vi "View param.vi"() -> ()   [LabVIEW 2019]
uses:
  Database/Progress.vi
panel:
  in  "PARNames":refnum<data-value>
  in  "PAR":refnum<data-value>
  in  "PARsh":refnum<data-value>
  in  "PAR_I":refnum<data-value>
  out "HandlingView":bool[](array[boolean])
  out "error out":errorcluster
  in  "n_elem2":i32
  in  "conninfo":T1={"host"="localhost", "port"="5432", "client_encoding"="WIN1251", "dbname"="system", "user"="postgres", "password"=""}
  in  "parameters 2":string[][](array[string])=[["H1.EB2.1.BT1", "H1.EB2.1.BT3", "H1.EB2.21.BT1", "H1.EB2.22.BT1", "H1.EB2.23.BT1", "H1.EB2.2.BT3", "H1.EB2.BP1", "H1.EB2.EP1.BF1", "H1.EB2.EP1.BT1", "H1.EB2.EP1.BT2", "H1.EB2.QN1", "H1.EP.BP1", "H1.GM2.1.BP1", "H1.GM2.1.HT1.BC1", "H1.GM2.1.HT1.BT1", "H1.GM2.1.QN1", "H1.GM2.2.BP1", "H1.GM2.2.QN1", "H1.GM2.2.QN2", "H1.GM2.2.QN3", "H1.HW2.BT1", "H1.HW2.BT2", "H1.HW2.BT3", "H1.HW2.BT4"]]
  in  "AOParamView":bool
  in  "DOParamView":bool
  out "n_modules":i32
  out "n_connect":i32
  in  "ModuleHandlingView":bool
  in  "ALRhandlingView":bool
  in  "AIParamView":bool
  out "tick out":u32=100 caption="Время цикла основной программы" min=5 max=500 step=1
  out "archiv AI period  out":u32=1000 caption="Период архивирования аналоговых параметров" min=1 max=100000 step=1
  out "archiv DI period  out":u32=1000 caption="Период архивирования дискретных параметров" min=1 max=100000 step=1
  out "modules read period out":u32=100 caption="Период обновления информации из модулей" min=1 max=100000 step=1
  out "Reread out":bool
  in  "modules read period":u32=500 caption="Период обновления информации из модулей" min=1 max=100000 step=1
  in  "ALR write":bool caption="запись аварийных сообщений"
  in  "DI write":bool caption="запись дискретных параметров"
  in  "AI write":bool caption="запись аналоговых параметров"
  in  "T_DB_write":u32(graph) caption="Время записи в БД"
  in  "archiv DI period":u32=1000 caption="Период архивирования дискретных параметров" min=1 max=100000 step=1
  in  "archiv AI period":u32=1000 caption="Период архивирования аналоговых параметров" min=1 max=100000 step=1
  in  "tick":u32=100 caption="Время цикла основной программы" min=5 max=500 step=1
  in  "n_elem":i32(c297)
  out "PAR progress":i32(slide) scale=0.0..100.0
  in  "Reread":bool
  out "units":string[](array[string])
  in  "AI_9":dbl min=1.0 max=10.0 step=1.0 format="%#.1f"
  in  "AI_10":dbl min=20.0 max=60.0 step=1.0 format="%#.1f"
  in  "AI_5":dbl min=10.0 max=1000.0 step=1.0 format="%#.1f"
  in  "AI_6":dbl min=10.0 max=10000.0 step=10.0 format="%#.1f"
  in  "AI_7":dbl min=1.0 max=10.0 step=1.0 format="%#.1f"
  in  "AI_8":dbl min=1.0 max=10.0 step=1.0 format="%#.1f"
  in  "AI_3":dbl min=1.0 max=50.0 step=1.0 format="%#.1f"
  in  "AI_4":dbl min=60000.0 max=300000.0 step=100.0 format="%#.1f"
  in  "AI_2":dbl min=50.0 max=60000.0 step=50.0 format="%#.1f"
  in  "AI_1":dbl min=50.0 max=60000.0 step=50.0 format="%#.1f"
  in  "ActivatePARView":bool
  out "n param":i32
  in  "parameters":string[](array[string])=["H1.EB2.1.BT1", "H1.EB2.1.BT3", "H1.EB2.21.BT1", "H1.EB2.22.BT1", "H1.EB2.23.BT1", "H1.EB2.2.BT3", "H1.EB2.BP1", "H1.EB2.EP1.BF1", "H1.EB2.EP1.BT1", "H1.EB2.EP1.BT2", "H1.EB2.QN1", "H1.EP.BP1", "H1.GM2.1.BP1", "H1.GM2.1.HT1.BC1", "H1.GM2.1.HT1.BT1", "H1.GM2.1.QN1", "H1.GM2.2.BP1", "H1.GM2.2.QN1", "H1.GM2.2.QN2", "H1.GM2.2.QN3", "H1.HW2.BT1", "H1.HW2.BT2", "H1.HW2.BT3", "H1.HW2.BT4"]
  out "This VI":refnum<vi>
  out "Names table":string[](array[string])=["температура нагревателя", "температура газа после ступени", "температура нагревателя", "температура нагревателя", "температура нагревателя", "температура газа после ступени", "давление газа перед нагревателем", "расход охлаждающей воды", "температура на входе", "температура на выходе", "регулятор расхода азота/тех газа", "давление охлаждающей воды на входе в теплообменник", "давление газа перед дозатором", "ток нагревателя", "температура нагревателя", "регулятор расхода азота/водорода (метана)", "давление газа перед дозатором", "регулятор расхода водорода (метана)", "регулятор природного газа", "дозатор жидкостный", "температура газа на входе в смеситель", "температура стенки смесителя 100 мм", "температура стенки смесителя 200 мм", "температура стенки смесителя на вводе CH4"]
  out "parameters1":string[](array[string])=["H1.EB2.1.BT1", "H1.EB2.1.BT3", "H1.EB2.21.BT1", "H1.EB2.22.BT1", "H1.EB2.23.BT1", "H1.EB2.2.BT3", "H1.EB2.BP1", "H1.EB2.EP1.BF1", "H1.EB2.EP1.BT1", "H1.EB2.EP1.BT2", "H1.EB2.QN1", "H1.EP.BP1", "H1.GM2.1.BP1", "H1.GM2.1.HT1.BC1", "H1.GM2.1.HT1.BT1", "H1.GM2.1.QN1", "H1.GM2.2.BP1", "H1.GM2.2.QN1", "H1.GM2.2.QN2", "H1.GM2.2.QN3", "H1.HW2.BT1", "H1.HW2.BT2", "H1.HW2.BT3", "H1.HW2.BT4"]
  # "mS"
  # "из"
  # "подключено"
  # "mS"
  # "mS"
  # "mS"
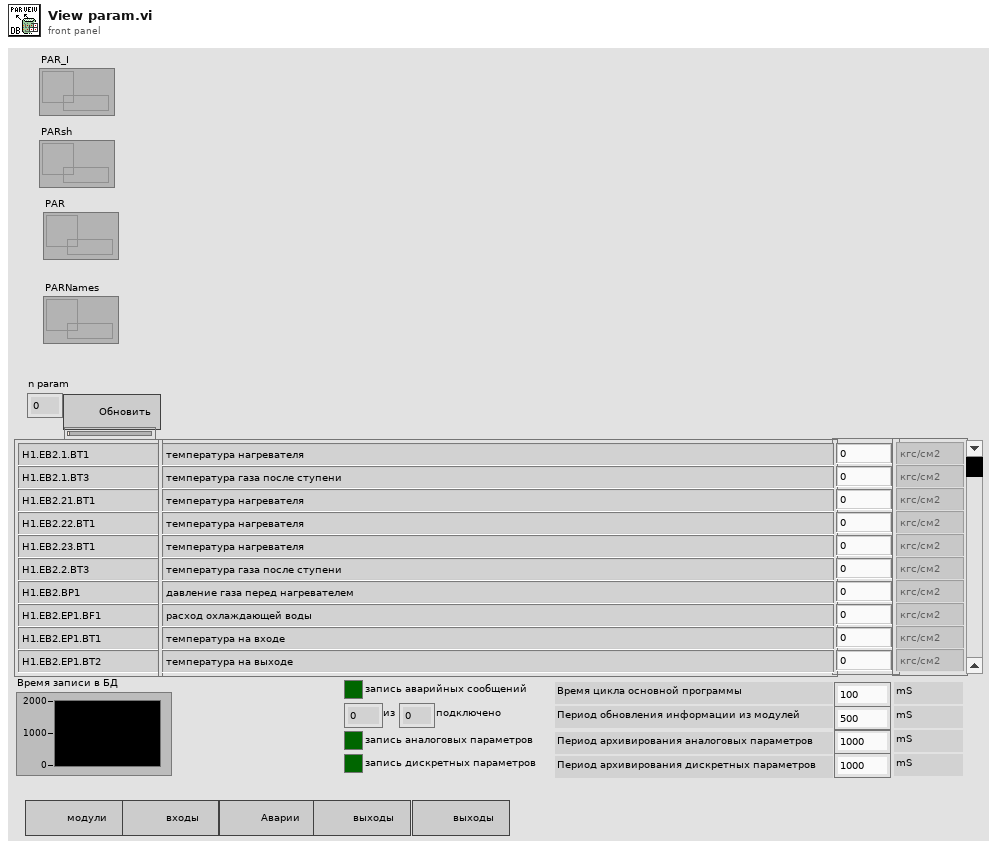
[diagram p1: front panel]
types:
  T1 = cluster{"host":string, "port":string, "client_encoding":string, "dbname":string, "user":string, "password":string}
  T2 = enum32{"Invalid", "Standard", "Closed", "Hidden", "Minimized", "Maximized"}
  T3 = enum16{"Start", "Connect", "Write enable", "IP address", "Errors"}
  T4 = enum16{"Init", "Read", "Read inputs", "Read outputs", "Write", "Write inputs"}
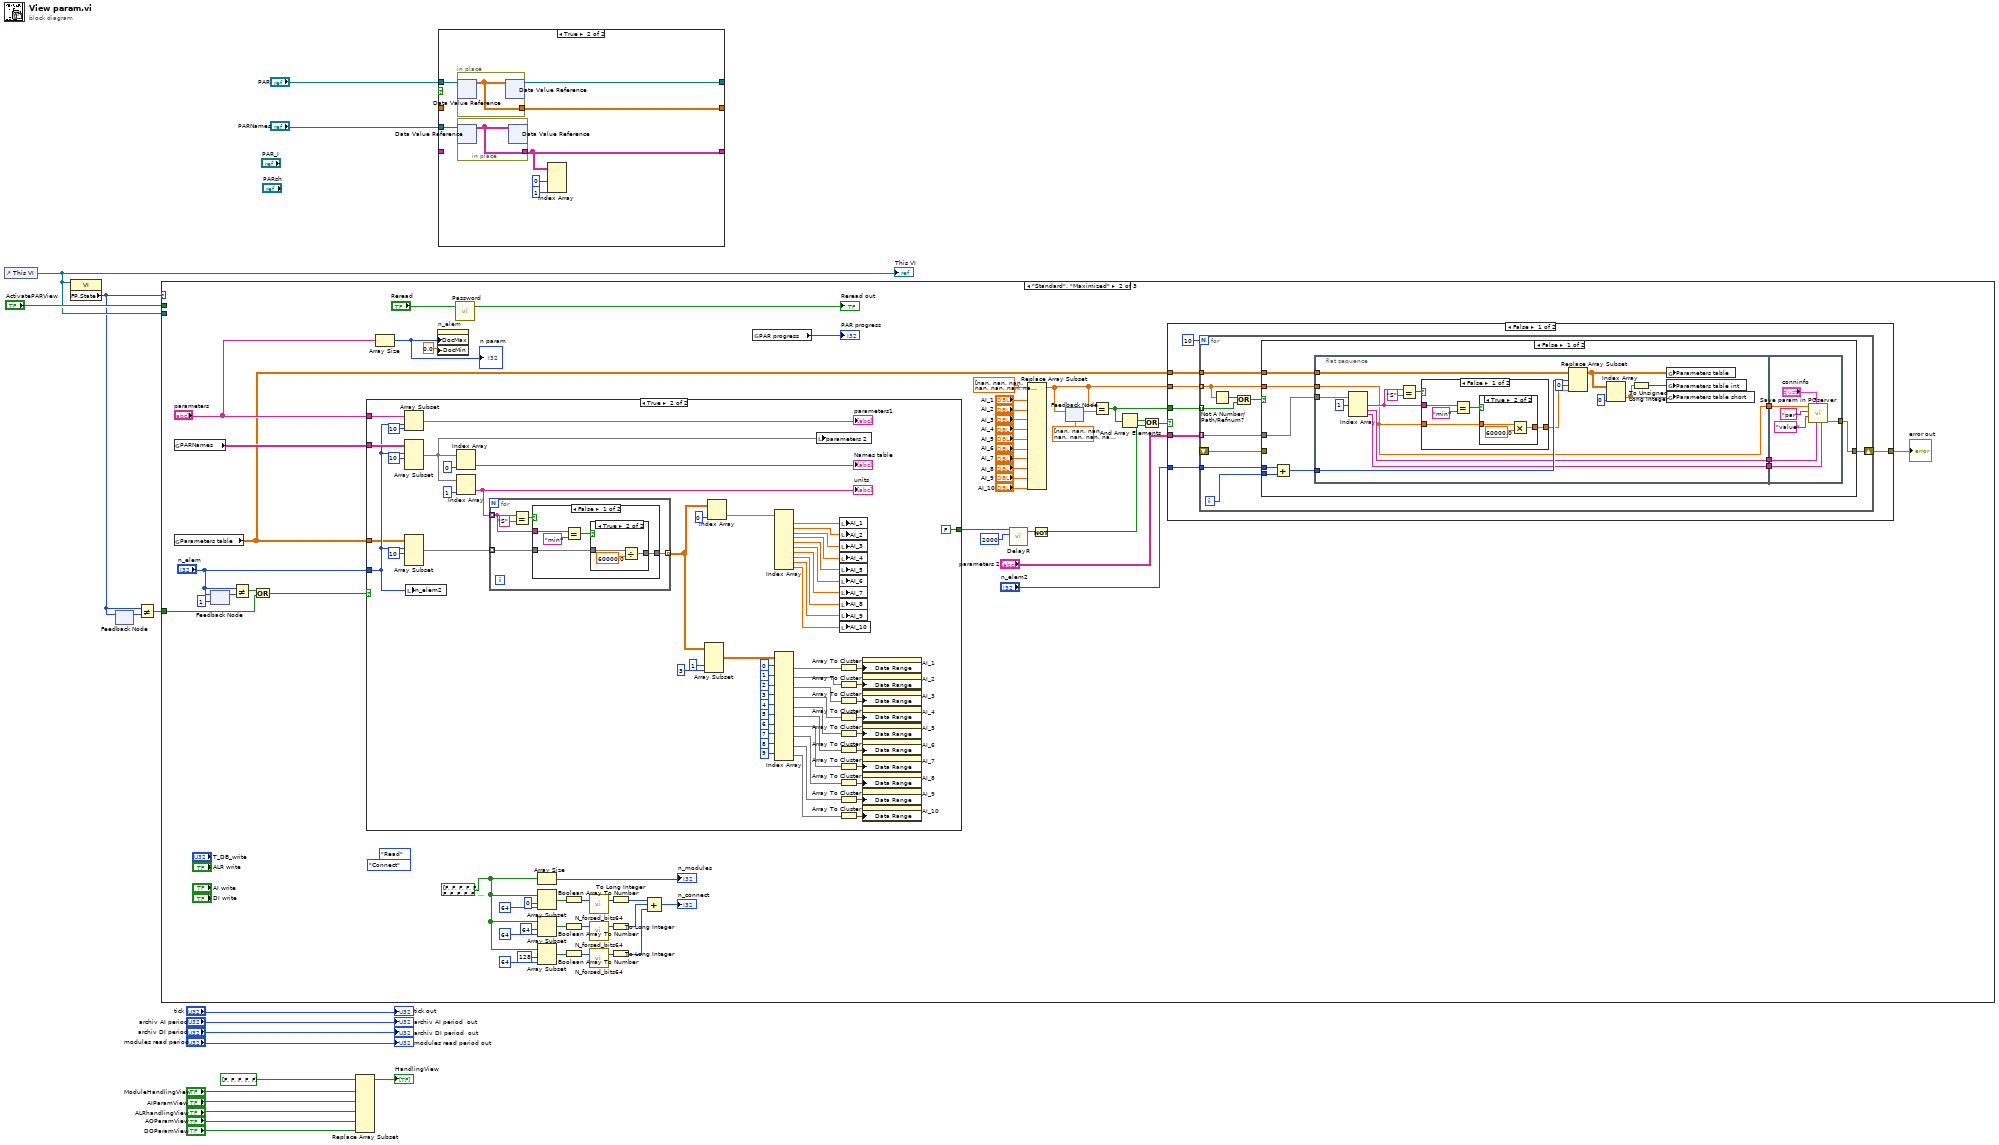
[diagram p0: block diagram]
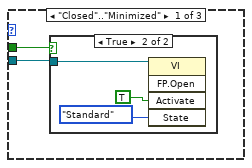
[diagram p3: hidden frame]
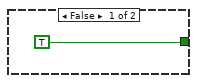
[diagram p5: hidden frame]
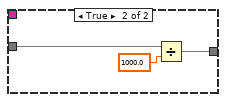
[diagram p7: hidden frame]
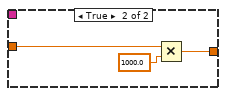
[diagram p9: hidden frame]
diagram:
  n1 = control-ref of="This VI"() -> (w17:refnum<vi>)
  "This VI" <- w17
  n2 = property class="VI"(reference=w17) -> ("FP.State"=w11:T2)  [unwired: 1 in, 2 out]
  n3 = feedback #1() -> (w12:T2)  [unwired: 1 in]
  n4 = feedback-in #1(w11) -> ()
  n5 = Not Equal?(x=w11, y=w12) -> (x != y?=w10:bool)
  n6 = case shown="\"Standard\", \"Maximized\"" w11 {
    tunnel: "ActivatePARView" -> [w20 _ _]
    tunnel: w17 -> [w19 _ _]
    tunnel: w10 -> [_ w24 _]
    frame "Closed".."Minimized" {
      n7 = case shown="True" w20 {
        tunnel: w19 -> [_ w21]
        frame False {
        }
        frame True {
          n8 = invoke class="VI" method="FP.Open"(reference=w21, "Activate"=TRUE ("Activate?"), "State"=T2."Standard") -> ()  [unwired: 2 in, 5 out]
        }
      }
    }
    frame "Standard", "Maximized" {
      w25 = bool[] [FALSE, FALSE, FALSE, FALSE, FALSE, FALSE, FALSE, FALSE, FALSE, FALSE, FALSE, FALSE, FALSE, FALSE, FALSE, FALSE, FALSE, FALSE, FALSE, FALSE, FALSE, FALSE, FALSE, FALSE, FALSE, FALSE, FALSE, FALSE, FALSE, FALSE, FALSE, FALSE, FALSE, FALSE, FALSE, FALSE, FALSE, FALSE, FALSE, FALSE, FALSE, FALSE, FALSE, FALSE, FALSE, FALSE, FALSE, FALSE, FALSE, FALSE, FALSE, FALSE, FALSE, FALSE, FALSE, FALSE, FALSE, FALSE, FALSE, FALSE, FALSE, FALSE, FALSE, FALSE, FALSE, FALSE, FALSE] ("connect")
      (unwired) T3."Connect" ("Table")
      (unwired) T4."Read" ("Function")
      n9 = global read "ep_parameters_190704.vi" "PARNames"() -> (w30:string[][])
      n10 = global read "ep_parameters_190704.vi" "Parameters table"() -> (w29:dbl[][])
      n11 = feedback #2(1 ("n_elem")) -> (w58:i32)
      n12 = feedback-in #2("n_elem") -> ()
      n13 = Not Equal?(x="n_elem", y=w58) -> (x != y?=w27:bool)
      n14 = Or(x=w27, y=w24) -> (x .or. y?=w26:bool)
      n15 = case shown="True" w26 {
        tunnel: w29 -> [_ w85]
        tunnel: w30 -> [_ w137]
        tunnel: "parameters" -> [_ w136]
        tunnel: "n_elem" -> [_ w88]
        tunnel: [TRUE FALSE] -> w34
        frame False {
        }
        frame True {
          n16 = Array Subset(array=w136, index=w88, length=10) -> (→"parameters1":string[])
          n17 = Array Subset(array=w137, index (row)=w88, length (row)=10 ("length")) -> (w99:string[][])  [unwired: 2 in]
          n18 = Array Subset(array=w85, index (row)=w88, length (row)=10 ("length")) -> (w120:dbl[][])  [unwired: 2 in]
          n19 = local write "n_elem2"(w88) -> ()
          n20 = Index Array(array=w99, index (col)=0 ("disabled index (col)")) -> (element=→"Names table":string[])  [unwired: 1 in]
          n21 = Index Array(array=w99, index (col)=1 ("disabled index (col)")) -> (element=w144:string[])  [unwired: 1 in]
          "units" <- w144
          n22 = for {
            tunnel: w144 -> [w145] mode=indexing
            tunnel: w120 -> [w148] mode=indexing
            tunnel: [w146] -> w87 mode=indexing
            n23 = Equal?(x=w145, y="S") -> (x = y?=w147:bool)
            n24 = case shown="False" w147 {
              tunnel: w148 -> [w154 w161]
              tunnel: [w153 w159] -> w146
              tunnel: w145 -> [w151 _]
              frame False {
                n25 = Equal?(x=w151, y="min") -> (x = y?=w152:bool)
                n26 = case shown="True" w152 {
                  tunnel: w154 -> [w155 w158]
                  tunnel: [w155 w156] -> w153
                  frame False {
                  }
                  frame True {
                    n27 = Divide(x=w158, y=60000.0) -> (x/y=w156:dbl[])
                  }
                }
              }
              frame True {
                n28 = Divide(x=w161, y=1000.0) -> (x/y=w159:dbl[])
              }
            }
          }
          n29 = Array Subset(array=w87, index (col)=1 ("length"), length (col)=3 ("length")) -> (w133:dbl[][])  [unwired: 2 in]
          n30 = Index Array(array=w87, index (col)=0 ("disabled index (col)")) -> (element=w86:dbl[])  [unwired: 1 in]
          n31 = Index Array(array=w86) -> (element #1=w98:dbl, element #2=w97:dbl, element #3=w96:dbl, element #4=w95:dbl, element #5=w94:dbl, element #6=w93:dbl, element #7=w92:dbl, element #8=w91:dbl, element #9=w90:dbl, element #10=w89:dbl)  [unwired: 10 in]
          n32 = Index Array(array=w133, index (row) #1=0 ("index (row)"), index (row) #2=1 ("index (row)"), index (row) #3=2 ("index (row)"), index (row) #4=3 ("index (row)"), index (row) #5=4 ("index (row)"), index (row) #6=5 ("index (row)"), index (row) #7=6 ("index (row)"), index (row) #8=7 ("index (row)"), index (row) #9=8 ("index (row)"), index (row) #10=9 ("index (row)")) -> (element #1=w118:dbl[], element #2=w116:dbl[], element #3=w114:dbl[], element #4=w113:dbl[], element #5=w110:dbl[], element #6=w109:dbl[], element #7=w107:dbl[], element #8=w105:dbl[], element #9=w104:dbl[], element #10=w103:dbl[])  [unwired: 10 in]
          n33 = local write "parameters 2"(w99) -> ()
          n34 = Array To Cluster(array=w118) -> (cluster=w119:cluster{"[0]":dbl, "[1]":dbl, "[2]":dbl})
          n35 = Array To Cluster(array=w116) -> (cluster=w117:cluster{"[0]":dbl, "[1]":dbl, "[2]":dbl})
          n36 = Array To Cluster(array=w114) -> (cluster=w111:cluster{"[0]":dbl, "[1]":dbl, "[2]":dbl})
          n37 = Array To Cluster(array=w113) -> (cluster=w112:cluster{"[0]":dbl, "[1]":dbl, "[2]":dbl})
          n38 = Array To Cluster(array=w110) -> (cluster=w100:cluster{"[0]":dbl, "[1]":dbl, "[2]":dbl})
          n39 = Array To Cluster(array=w109) -> (cluster=w108:cluster{"[0]":dbl, "[1]":dbl, "[2]":dbl})
          n40 = Array To Cluster(array=w107) -> (cluster=w106:cluster{"[0]":dbl, "[1]":dbl, "[2]":dbl})
          n41 = Array To Cluster(array=w105) -> (cluster=w102:cluster{"[0]":dbl, "[1]":dbl, "[2]":dbl})
          n42 = Array To Cluster(array=w104) -> (cluster=w101:cluster{"[0]":dbl, "[1]":dbl, "[2]":dbl})
          n43 = Array To Cluster(array=w103) -> (cluster=w115:cluster{"[0]":dbl, "[1]":dbl, "[2]":dbl})
          n44 = local write "AI_1"(w98) -> ()
          n45 = local write "AI_2"(w97) -> ()
          n46 = local write "AI_3"(w96) -> ()
          n47 = local write "AI_4"(w95) -> ()
          n48 = local write "AI_5"(w94) -> ()
          n49 = local write "AI_6"(w93) -> ()
          n50 = local write "AI_7"(w92) -> ()
          n51 = local write "AI_8"(w91) -> ()
          n52 = local write "AI_9"(w90) -> ()
          n53 = local write "AI_10"(w89) -> ()
          n54 = property on="AI_1" class="DigNum (strict)"("Data Range"=w119) -> ()  [unwired: 2 in, 2 out]
          n55 = property on="AI_2" class="DigNum (strict)"("Data Range"=w117) -> ()  [unwired: 2 in, 2 out]
          n56 = property on="AI_3" class="DigNum (strict)"("Data Range"=w111) -> ()  [unwired: 2 in, 2 out]
          n57 = property on="AI_4" class="DigNum (strict)"("Data Range"=w112) -> ()  [unwired: 2 in, 2 out]
          n58 = property on="AI_5" class="DigNum (strict)"("Data Range"=w100) -> ()  [unwired: 2 in, 2 out]
          n59 = property on="AI_6" class="DigNum (strict)"("Data Range"=w108) -> ()  [unwired: 2 in, 2 out]
          n60 = property on="AI_7" class="DigNum (strict)"("Data Range"=w106) -> ()  [unwired: 2 in, 2 out]
          n61 = property on="AI_8" class="DigNum (strict)"("Data Range"=w102) -> ()  [unwired: 2 in, 2 out]
          n62 = property on="AI_9" class="DigNum (strict)"("Data Range"=w101) -> ()  [unwired: 2 in, 2 out]
          n63 = property on="AI_10" class="DigNum (strict)"("Data Range"=w115) -> ()  [unwired: 2 in, 2 out]
        }
      }
      n64 = Array Size(array="parameters") -> (size(s)=w56:i32)
      "n param" <- w56
      n65 = property on="n_elem" class="Scroll (strict)"("DocMax"=w56, "DocMin"=0.0 ("Doc Min")) -> ()  [unwired: 2 in, 2 out]
      n66 = call "Password.vi"("ActivatePASSWView"="Reread") -> ("enable"=→"Reread out":bool)  [unwired: 1 in, 1 out]
      n67 = Array Size(array=w25) -> (size(s)=→"n_modules":i32)
      n68 = Array Subset(array=w25, index=0, length=64) -> (w65:bool[])
      n69 = Array Subset(array=w25, index=64, length=64) -> (w71:bool[])
      n70 = Array Subset(array=w25, index=128, length=64) -> (w70:bool[])
      n71 = Boolean Array To Number(Boolean array=w65) -> (number=w72:u64)
      n72 = Boolean Array To Number(Boolean array=w71) -> (number=w73:u64)
      n73 = Boolean Array To Number(Boolean array=w70) -> (number=w74:u64)
      n74 = call "N_forsed_bits64.vi"("IN"=w72) -> ("N_forsed_bits"=w75:u64)  [unwired: 2 in]
      n75 = call "N_forsed_bits64.vi"("IN"=w73) -> ("N_forsed_bits"=w79:u64)  [unwired: 2 in]
      n76 = call "N_forsed_bits64.vi"("IN"=w74) -> ("N_forsed_bits"=w77:u64)  [unwired: 2 in]
      n77 = To Long Integer(number=w75) -> (32bit integer=w76:i32)
      n78 = To Long Integer(number=w79) -> (32bit integer=w80:i32)
      n79 = To Long Integer(number=w77) -> (32bit integer=w78:i32)
      n80 = Compound Arithmetic op=ADD(w76, w80, w78) -> (→"n_connect":i32)
      n81 = global read "Progress.vi" "PAR progress"() -> (→"PAR progress":i32)
      n82 = call "DelayR.vi"("DelayOn"=u32 2000 ("DelayOff"), "In"=w34) -> ("Out"=w33:bool)  [unwired: 2 in, 1 out]
      n83 = Replace Array Subset(array=dbl[] [nan, nan, nan, nan, nan, nan, nan, nan, nan, nan] ("Parameters table"), new element #1="AI_1", new element #2="AI_2", new element #3="AI_3", new element #4="AI_4", new element #5="AI_5", new element #6="AI_6", new element #7="AI_7", new element #8="AI_8", new element #9="AI_9", new element #10="AI_10") -> (w37:dbl[])  [unwired: 10 in]
      n84 = Not(x=w33) -> (.not. x?=w31:bool)
      n85 = feedback-in #3(w37) -> ()
      n86 = feedback #3(dbl[] [nan, nan, nan, nan, nan, nan, nan, nan, nan, nan] ("Parameters table")) -> (w35:dbl[])
      n87 = Equal?(x=w37, y=w35) -> (x = y?=w40:bool[])
      n88 = And Array Elements(Boolean array=w40) -> (logical AND=w39:bool)
      n89 = Or(x=w39, y=w31) -> (x .or. y?=w38:bool)
      n90 = case shown="False" w38 {
        tunnel: "parameters 2" -> [w167 _]
        tunnel: "n_elem2" -> [w166 _]
        tunnel: [w165 _] -> w51
        tunnel: w29 -> [w164 _]
        tunnel: w37 -> [w162 _]
        tunnel: w40 -> [w163 _]
        frame False {
          n91 = for {
            N: 10 -> [_]
            tunnel: w167 -> [w178] mode=indexing
            tunnel: w166 -> [w177]
            tunnel: w164 -> [w176]
            tunnel: w162 -> [w172] mode=indexing
            tunnel: w163 -> [w169] mode=indexing
            shift-right: [w175] -> w165
            shift-left: _ -> [w173]
            i -> [w174]
            n92 = Not A Number/Path/Refnum?(number/path/refnum=w172) -> (NaN/Path/Refnum?=w170:bool)
            n93 = Or(x=w170, y=w169) -> (x .or. y?=w171:bool)
            n94 = case shown="False" w171 {
              tunnel: w178 -> [w188 _]
              tunnel: w177 -> [w186 _]
              tunnel: w176 -> [w187 _]
              tunnel: [w184 w224] -> w175
              tunnel: w172 -> [w180 _]
              tunnel: w174 -> [w179 _]
              tunnel: w173 -> [_ w224]
              frame False {
                n95 = Add(x=w186, y=w179) -> (x+y=w185:i32)
                n96 = flat-sequence {
                  tunnel: w188 -> [w198]
                  tunnel: w187 -> [w204]
                  tunnel: w185 -> [w203]
                  tunnel: w180 -> [w189]
                  tunnel: [w189] -> w183
                  tunnel: [w197] -> w182
                  tunnel: [w196] -> w181
                  tunnel: [w221] -> w184
                  tunnel: w183 -> [w222]
                  tunnel: w182 -> [w219]
                  tunnel: w181 -> [w218]
                  frame #0 {
                    n97 = Index Array(array=w198, index #1=1 ("disabled index (col)")) -> (element #1=w190:string, element #2=w197:string, element #3=w196:string)  [unwired: 2 in]
                    n98 = Equal?(x=w190, y="S") -> (x = y?=w191:bool)
                    n99 = case shown="False" w191 {
                      tunnel: w189 -> [w209 w216]
                      tunnel: [w208 w214] -> w192
                      tunnel: w190 -> [w206 _]
                      frame False {
                        n100 = Equal?(x=w206, y="min") -> (x = y?=w207:bool)
                        n101 = case shown="True" w207 {
                          tunnel: w209 -> [w210 w213]
                          tunnel: [w210 w211] -> w208
                          frame False {
                          }
                          frame True {
                            n102 = Multiply(x=w213, y=60000.0) -> (x*y=w211:dbl)
                          }
                        }
                      }
                      frame True {
                        n103 = Multiply(x=w216, y=1000.0) -> (x*y=w214:dbl)
                      }
                    }
                    n104 = Replace Array Subset(array=w204, new element=w192, index (row)=w203, index (col)=0 ("disabled index (col)")) -> (w193:dbl[][])
                    n105 = Index Array(array=w193, index (col)=0 ("disabled index (col)")) -> (element=w194:dbl[])  [unwired: 1 in]
                    n106 = To Unsigned Long Integer(number=w194) -> (unsigned 32bit integer=w195:u32[])
                    n107 = global write "ep_parameters_190704.vi" "Parameters table"(w193) -> ()
                    n108 = global write "ep_parameters_190704.vi" "Parameters table int"(w195) -> ()
                    n109 = global write "ep_parameters_190704.vi" "Parameters table short"(w194) -> ()
                  }
                  frame #1 {
                    n110 = call "Save param in PGserver.vi"("Param row name 2"=w218, "Param row name1"=w219, "conninfo"="conninfo", "Param column Name"="value" ("Param Table"), "Param Table"="par", "Parameter"=w222) -> ("error out"=w221:errorcluster)  [unwired: 5 in]
                  }
                }
              }
              frame True {
              }
            }
          }
        }
        frame True {
        }
      }
      "error out" <- w51
    }
    frame "Invalid", Default {
    }
  }
  n111 = Replace Array Subset(array=bool[] [FALSE, FALSE, FALSE, FALSE, FALSE], new element #1="ModuleHandlingView", new element #2="AIParamView", new element #3="ALRhandlingView", new element #4="AOParamView", new element #5="DOParamView") -> (→"HandlingView":bool[])  [unwired: 5 in]
  n112 = case shown="True" {
    selector: _ -> [_ _]
    tunnel: [w226 w233] -> _
    tunnel: [w227 w234] -> _
    tunnel: "PAR" -> [w225 w230]
    tunnel: "PARNames" -> [_ w229]
    tunnel: _ -> [w227 _]
    tunnel: _ -> [w226 _]
    tunnel: [w225 w228] -> _
    frame False {
    }
    frame True {
      n113 = in-place {
        in-place-border: [w236] -> w234
        n114 = in-place-dvr #4(w230) -> (w236:dbl[][])  [unwired: 1 out]
        n115 = in-place-dvr #4(w236) -> (w228:refnum<data-value>)  [unwired: 1 out]
      }
      n116 = in-place {
        in-place-border: [w235] -> w233
        n117 = in-place-dvr #5(w229) -> (w235:string[][])  [unwired: 1 out]
        n118 = in-place-dvr #5(w235) -> ()  [unwired: 2 out]
      }
      n119 = Index Array(array=w233, index (col) #1=0 ("index (row)"), index (col) #2=1 ("index (row)")) -> ()  [unwired: 2 in, 2 out]
    }
  }
  "tick out" <- "tick"
  "archiv AI period  out" <- "archiv AI period"
  "archiv DI period  out" <- "archiv DI period"
  "modules read period out" <- "modules read period"
